vi "change tab size.vi"(11 "Tab Ref In":refnum<vi>) -> ()   [LabVIEW 2012]
panel:
  in  "Stop Button":bool
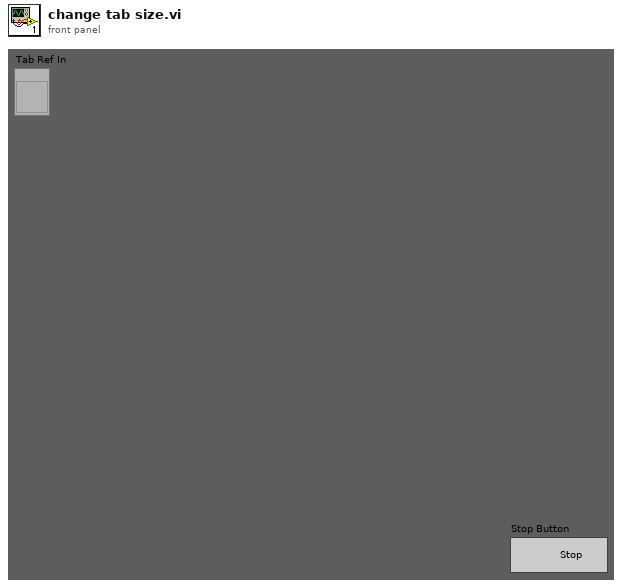
[diagram p1: front panel]
types:
  T1 = typedef "LVBoundsTypeDef.ctl" = cluster{"Width":u32, "Height":u32}
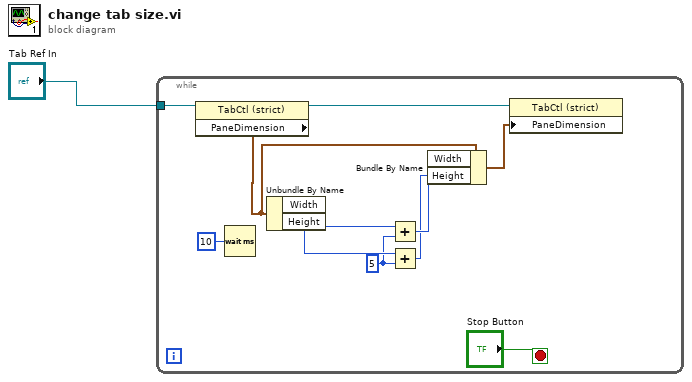
[diagram p0: block diagram]
diagram:
  n1 = while {
    tunnel: "Tab Ref In" -> [w4]
    stop <- "Stop Button" stop-if-true
    w6 = 5 ("y")
    n2 = property class="TabCtl (strict)"(reference=w4) -> (reference out=w3:refnum<vi>, "PaneDimension"=w5:T1)  [unwired: 1 in, 1 out]
    n3 = Wait (ms)(milliseconds to wait=u32 10) -> ()  [unwired: 1 out]
    n4 = Unbundle By Name(w5) -> ("Width"=w11:u32, "Height"=w10:u32)
    n5 = Add(x=w11, y=w6) -> (x+y=w8:u32)
    n6 = Add(x=w10, y=w6) -> (x+y=w7:u32)
    n7 = Bundle By Name(cluster=w5, "Width"=w8, "Height"=w7) -> (w2:T1)
    n8 = property class="TabCtl (strict)"(reference=w3, "PaneDimension"=w2) -> ()  [unwired: 1 in, 2 out]
  }
